vi "Setup subWorker - Cam UI.vi"(8 "error in":errorcluster, 11 "Camera detection in":refnum<class "Camera detection.lvclass">) -> (0 "error out":errorcluster, 3 "Camera detection out":refnum<class "Camera detection.lvclass">)   [LabVIEW 2026, in "Camera detection.lvclass"]
doc: "This VI sets up the framework parameters of a statically-linked subWorker."
uses:
  Camera detection.lvclass
  Camera detection.lvclass/Camera detection.ctl
  C:/Program Files/National Instruments/LabVIEW 2026/vi.lib/addons/_Workers/Library/Classes/Worker/Worker.lvclass
  C:/Program Files/National Instruments/LabVIEW 2026/vi.lib/addons/_Workers/Library/Classes/Workers Object/Workers Object.lvclass
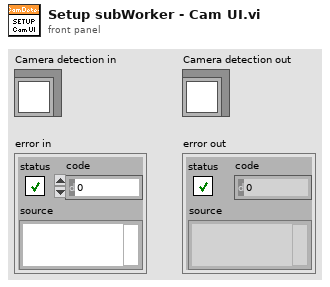
[diagram p1: front panel]
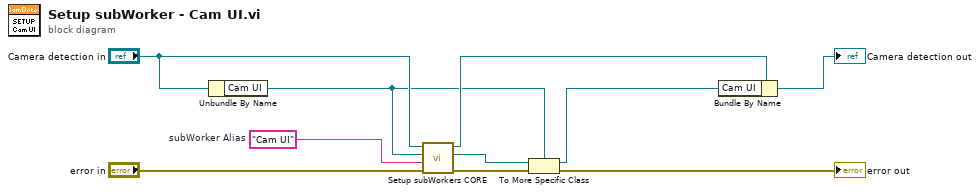
[diagram p0: block diagram]
diagram:
  w6 = "Cam UI"  # subWorker Alias
  n1 = Unbundle By Name("Camera detection in") -> ("Cam UI"=w3:refnum<class "Caméra UI.lvclass">)
  n2 = call-dynamic "Setup subWorkers CORE.vi"("error in"="error in", "subWorker Alias"=w6, "subWorker"=w3, "Worker"="Camera detection in") -> ("error out"=w5:errorcluster, "subWorker out"=w1:refnum<class "Worker.lvclass">, "Worker out"=w8:refnum<class "Camera detection.lvclass">)  [unwired: 5 in]
  n3 = To More Specific Class(target class=w3, reference=w1, error in=w5) -> (specific class reference=w2:refnum<class "Caméra UI.lvclass">, error out=→"error out":errorcluster)
  n4 = Bundle By Name(cluster=w8, "Cam UI"=w2) -> (→"Camera detection out":refnum<class "Camera detection.lvclass">)
